vi "MainAmmeterComm.vi"() -> ()   [LabVIEW 2010]
uses:
  BaudRate.ctl
  VarableID.ctl
panel:
  out "Legend:Plot Minimum":u32
  in  "视在功率":bool=TRUE
  in  "功率因数":bool=TRUE
  in  "电压":bool=TRUE
  in  "电流":bool=TRUE
  in  "退出系统":bool
  in  "软件使用说明":bool
  in  "启动采集":bool=TRUE
  in  "baud rate":T1=2400 caption="波特率" items=["1200"=1200, "2400"=2400, "4800"=4800, "9600"=9600, "19200"=19200, "38400"=38400, "115200"=115200, ""=0]
  out "测量变量显示":dbl[][](graph)
  # "智能电表信息采集系统"
  # "信号采集选项"
  # "端口参数设置"
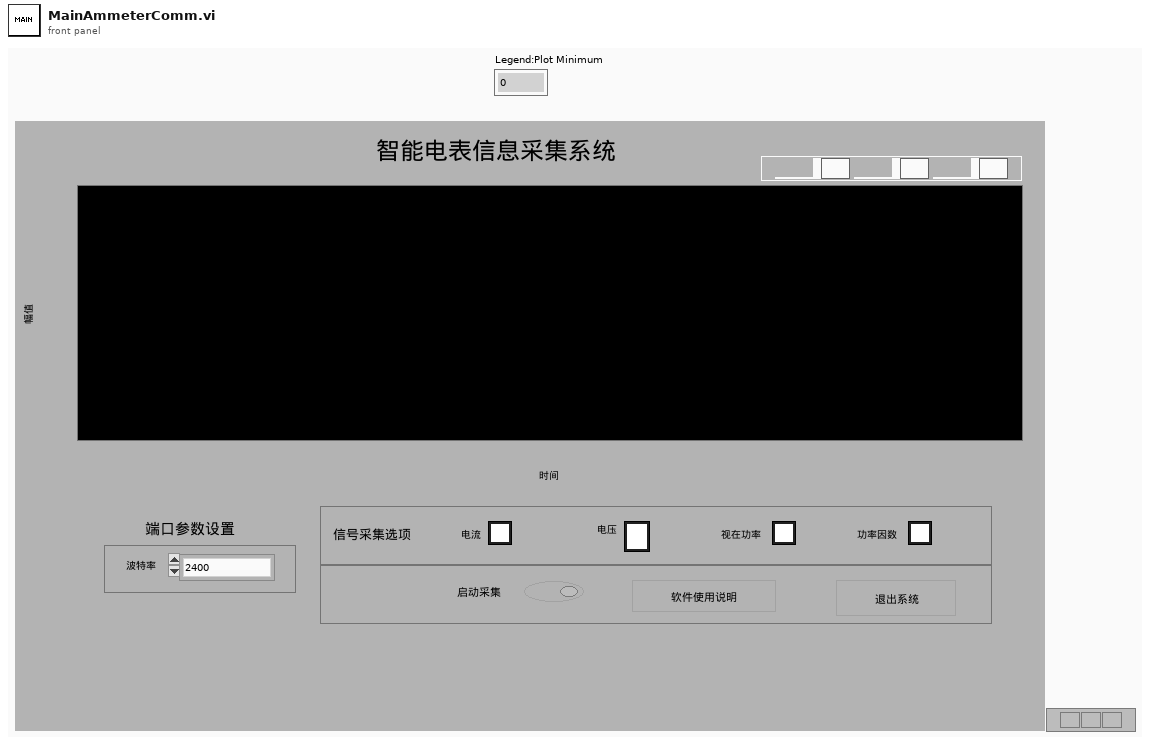
[diagram p1: front panel]
types:
  T1 = typedef "BaudRate.ctl" = u64
  T2 = typedef "OutputDataFormat.ctl" = cluster{"property":string, "dataIdentity":string, "value":string, "address":string}
  T3 = typedef "VarableID.ctl" = enum16{"current", "voltage", "power", "PF"}
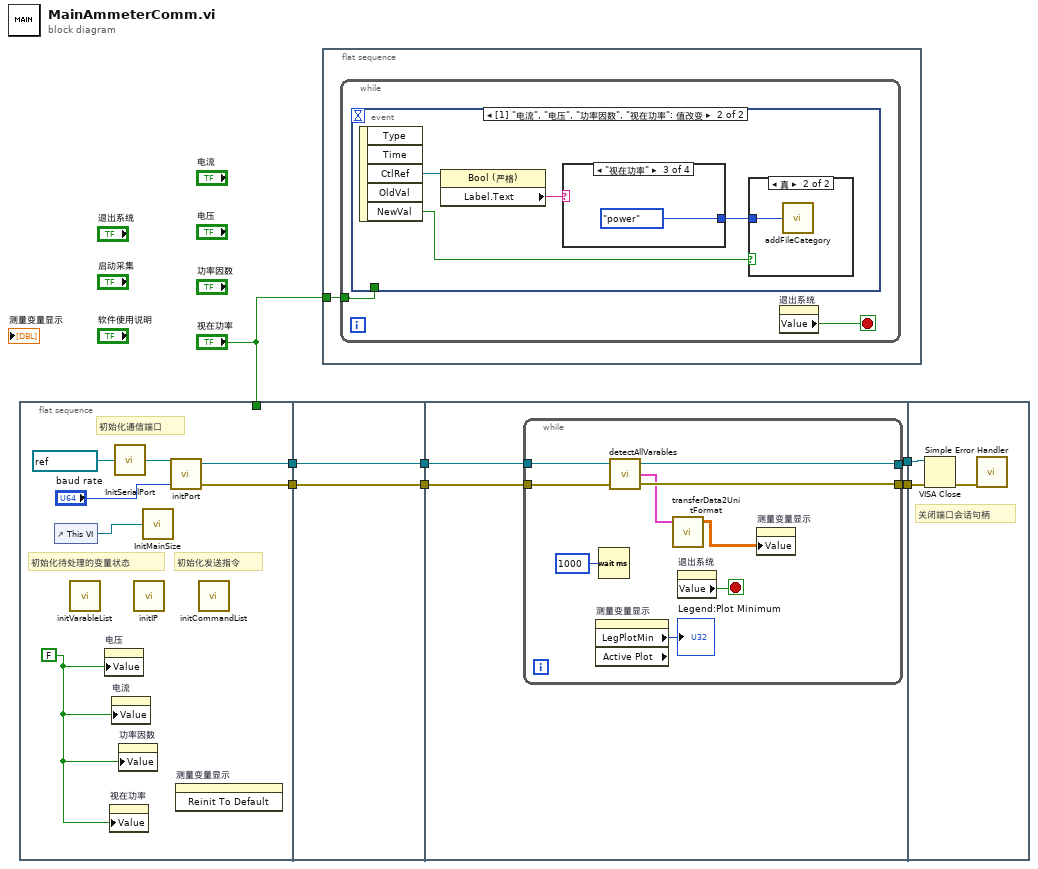
[diagram p0: block diagram]
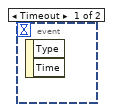
[diagram p2: hidden frame]
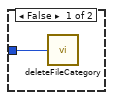
[diagram p3: hidden frame]
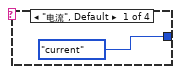
[diagram p4: hidden frame]
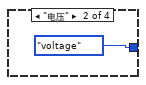
[diagram p5: hidden frame]
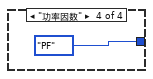
[diagram p6: hidden frame]
diagram:
  n1 = flat-sequence {
    tunnel: [w12] -> w3
    tunnel: "视在功率" -> [_]
    tunnel: [w13] -> w2
    tunnel: [w16] -> w4
    tunnel: w3 -> [w15]
    tunnel: w2 -> [w16]
    tunnel: [w15] -> w1
    tunnel: w4 -> [w20]
    tunnel: [w19] -> w7
    tunnel: [w18] -> w6
    tunnel: w1 -> [w17]
    tunnel: w7 -> [w31]
    tunnel: w6 -> [w30]
    frame #0 {
      w8 = FALSE
      # "初始化发送指令"
      # "初始化通信端口"
      # "初始化待处理的变量状态"
      n2 = control-ref of="This VI"() -> (w9:refnum<vi>)
      n3 = call "initVarableList.vi"() -> ()  [unwired: 12 in]
      n4 = property on="电压" class="Bool (严格)"("Value"=w8) -> ()  [unwired: 2 in, 2 out]
      n5 = property on="视在功率" class="Bool (严格)"("Value"=w8) -> ()  [unwired: 2 in, 2 out]
      n6 = property on="电流" class="Bool (严格)"("Value"=w8) -> ()  [unwired: 2 in, 2 out]
      n7 = call "InitSerialPort.vi"("default resource name"=refnum<visa-resource-name> "COM7" ("Port")) -> ("VISA resource name out"=w10:refnum<visa-resource-name>)
      n8 = property on="功率因数" class="Bool (严格)"("Value"=w8) -> ()  [unwired: 2 in, 2 out]
      n9 = call "initIP.vi"() -> ()  [unwired: 12 in]
      n10 = call "InitMainSize.vi"("VI Refnum In"=w9) -> ()  [unwired: 1 out]
      n11 = call "initPort.vi"("baud rate"="baud rate", "VISA resource name"=w10) -> ("error out"=w13:errorcluster, "reference out"=w12:refnum<visa-resource-name>)  [unwired: 2 in]
      n12 = invoke on="测量变量显示" class="WFChart (严格)" method="Reinit To Default"() -> ()  [unwired: 3 in, 3 out]
      n13 = call "initCommandList.vi"() -> ()  [unwired: 12 in]
    }
    frame #1 {
    }
    frame #2 {
      n14 = while {
        tunnel: w20 -> [w25]
        tunnel: [w26] -> w19
        tunnel: [w28] -> w18
        tunnel: w17 -> [w27]
        stop <- w29 stop-if-true
        n15 = property on="测量变量显示" class="WFChart (严格)" props=["LegPlotMin", "Active Plot"]() -> ("LegPlotMin"=→"Legend:Plot Minimum":u32)  [unwired: 2 in, 3 out]
        n16 = Wait (ms)(milliseconds to wait=u32 1000) -> ()  [unwired: 1 out]
        n17 = call "detectAllVarables.vi"("error in (no error)"=w25, "VISA resource name"=w27) -> ("error out"=w28:errorcluster, "Data"=w24:T2[], "VISA resource name 2"=w26:refnum<visa-resource-name>)  [unwired: 1 in]
        n18 = call "transferData2UnitFormat.vi"("Data"=w24) -> ("display"=w23:dbl[][])  [unwired: 4 in]
        n19 = property on="退出系统" class="Bool (严格)"() -> ("Value"=w29:bool)  [unwired: 2 in, 2 out]
        n20 = property on="测量变量显示" class="WFChart (严格)"("Value"=w23) -> ()  [unwired: 2 in, 2 out]
      }
    }
    frame #3 {
      # "关闭端口会话句柄"
      n21 = VISA Close(VISA resource name=w31, error in (no error)=w30) -> (error out=w32:errorcluster)
      n22 = call <vilib>:"Simple Error Handler.vi"("error in (no error)"=w32) -> ()  [unwired: 1 in, 8 out]
    }
  }
  n23 = flat-sequence {
    tunnel: "视在功率" -> [w33]
    frame #0 {
      n24 = while {
        tunnel: w33 -> [w35]
        stop <- w34 stop-if-true
        n25 = event shown="[1] \"电流\", \"电压\", \"功率因数\", \"视在功率\": 值改变" {
          selector: _ -> [_ _]
          dyn-events: _ -> [_ _]
          timeout: _ -> [_ _]
          tunnel: w35 -> [_ _]
          event Timeout {
            n26 = event-data() -> ()  [unwired: 1 in, 2 out]
          }
          event "电流", "电压", "功率因数", "视在功率": Value Change {
            n27 = event-data() -> ("CtlRef"=w36:refnum<vi>, "NewVal"=w37:bool)  [unwired: 1 in, 3 out]
            n28 = property class="Bool (严格)"(reference=w36) -> ("Label.Text"=w39:string)  [unwired: 1 in, 2 out]
            n29 = case shown="\"视在功率\"" w39 {
              tunnel: [VarableID."current" ("VarableID") VarableID."voltage" ("VarableID") VarableID."power" ("VarableID") VarableID."PF" ("VarableID")] -> w38
              frame "电流", Default {
              }
              frame "电压" {
              }
              frame "视在功率" {
              }
              frame "功率因数" {
              }
            }
            n30 = case shown="真" w37 {
              tunnel: w38 -> [w40 w41]
              frame False {
                n31 = call "deleteFileCategory.vi"("VarableID"=w40) -> ()  [unwired: 1 in]
              }
              frame True {
                n32 = call "addFileCategory.vi"("VarableID"=w41) -> ()  [unwired: 1 in]
              }
            }
          }
        }
        n33 = property on="退出系统" class="Bool (严格)"() -> ("Value"=w34:bool)  [unwired: 2 in, 2 out]
      }
    }
  }
